vi "slope.vi"() -> ()   [LabVIEW 2022 SP3]
panel:
  out "Slope":dbl
  in  "Y2":dbl
  in  "Y1":dbl
  in  "X2":dbl
  in  "X1":dbl
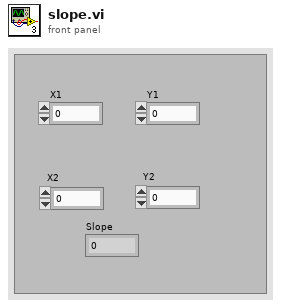
[diagram p1: front panel]
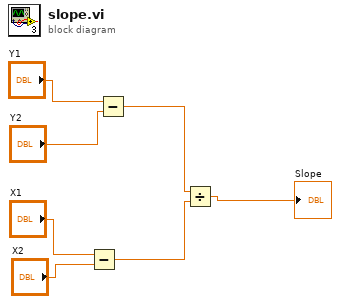
[diagram p0: block diagram]
diagram:
  n1 = Subtract(x="X1", y="X2") -> (x-y=w2:dbl)
  n2 = Subtract(x="Y1", y="Y2") -> (x-y=w3:dbl)
  n3 = Divide(x=w3, y=w2) -> (x/y=→"Slope":dbl)
